vi "复位F620.vi"() -> ()   [LabVIEW 2014]
uses:
  <vilib>/Modbus/master/Create Master Instance (Serial).vi
  <vilib>/Modbus/master/Modbus Master.lvclass
panel:
  out "error out":errorcluster caption="错误输出"
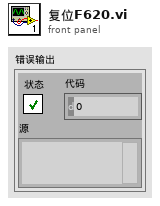
[diagram p1: front panel]
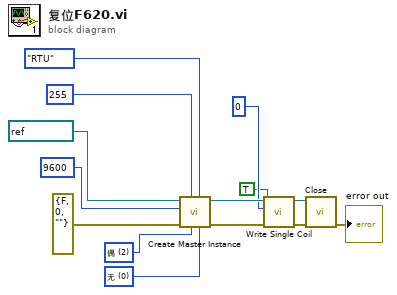
[diagram p0: block diagram]
diagram:
  w12 = u16 2 items=["无", "奇", "偶"] ("parity (Even)")
  w14 = u16 0 items=["无", "XON/XOFF", "RTS/CTS", "XON/XOFF & RTS/CTS", "DTR/DSR", "XON/XOFF & DTR/DSR"] ("flow control (None)")
  n1 = call-poly <vilib>:"Create Master Instance.vi"("flow control (None)"=w14, "serial type"=enum16{"RTU", "ASCII"}."RTU", "parity (Even)"=w12, "unit ID"=u8 255, "error in (no error)"=errorcluster {"status"=FALSE, "code"=0, "source"=""}, "baud rate (9600)"=u32 9600, "VISA resource name"=refnum<visa-resource-name> "COM6") -> ("error out"=w6:errorcluster, "serial master instance"=w7:refnum<class "Modbus Master.lvclass">)  [unwired: 3 in]
  n2 = call-dynamic "Write Single Coil.vi"("error in (no error)"=w6, "coil value"=TRUE, "address"=u16 0, "Modbus master in"=w7) -> ("error out"=w3:errorcluster, "Modbus master out"=w4:refnum<class "Modbus Master.lvclass">)  [unwired: 6 in]
  n3 = call-dynamic "Close.vi"("error in (no error)"=w3, "Modbus master in"=w4) -> ("error out"=→"error out":errorcluster)  [unwired: 9 in]
